vi "Get Timestamp.vi"(8 "error in (no error)":errorcluster, 9 "Data Type (default value)":timestamp, 10 "Offset":i32, 11 "JSON":string) -> (0 "error out":errorcluster, 1 "Timestamp":timestamp, 2 "Offset past match":i32)   [LabVIEW 2017, in "JSONtext.lvlib"]
uses:
  JSONtext.lvlib
  Parsing/Advance past String.vi
  String Subset.vi
  Strip Quotes and Unescape.vi
  Get Number Text.vi
  Parsing/NaN or null to Integer ERROR.vi
  Parsing/Advance past Number.vi
  <vilib>/Utility/error.llb/Error Cluster From Error Code.vi
  Parsing/Parsing Error.vi
  Unescape JSON string.vi
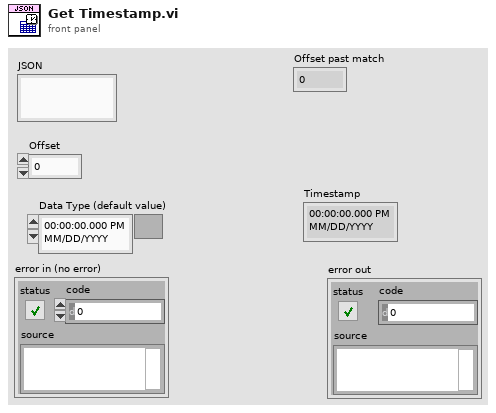
[diagram p1: front panel]
types:
  T1 = typedef "JSONtext.lvlib/Parsing State.ctl" = enum16{"Parser Error", "Object", "Array", "String", "Number/Other", "Leading Whitespace", "Object end", "Array end", "Value end"}
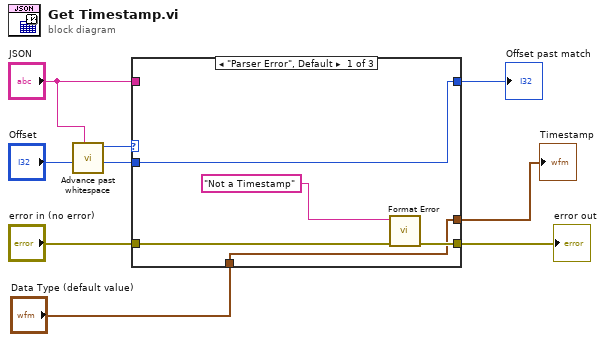
[diagram p0: block diagram]
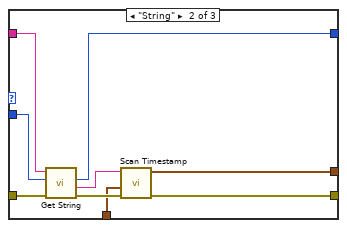
[diagram p2: hidden frame]
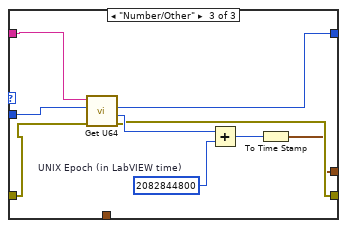
[diagram p3: hidden frame]
diagram:
  n1 = call "Advance past whitespace.vi"("JSON"="JSON", "Offset"="Offset") -> ("Offset of first non-whitespace"=w3:i32, "Parser State"=w2:T1)  [unwired: 8 in]
  n2 = case shown="\"Parser Error\", Default" w2 {
    tunnel: "error in (no error)" -> [w13 w23 w27]
    tunnel: [w11 w20 w25] -> w8
    tunnel: [w14 w19 w26] -> w7
    tunnel: [w12 w18 w24] -> w6
    tunnel: "JSON" -> [_ w17 w32]
    tunnel: w3 -> [w12 w16 w31]
    tunnel: "Data Type (default value)" -> [w11 w15 _]
    frame "Parser Error", Default {
      n3 = call "Format Error.vi"("error in (no error)"=w13, "error message"="Not a Timestamp" ("format string")) -> ("error out"=w14:errorcluster)  [unwired: 9 in]
    }
    frame "String" {
      n4 = call "Get String.vi"("error in (no error)"=w23, "Offset"=w16, "JSON"=w17) -> ("error out"=w22:errorcluster, "String"=w21:string, "Offset past match"=w18:i32)  [unwired: 6 in]
      n5 = call "Scan Timestamp.vi"("error in (no error)"=w22, "default value"=w15, "String"=w21) -> ("error out"=w19:errorcluster, "Timestamp"=w20:timestamp)  [unwired: 7 in]
    }
    frame "Number/Other" {
      w30 = i64 2082844800  # UNIX Epoch (in LabVIEW time)
      n6 = call "Get U64.vi"("error in (no error)"=w27, "Offset"=w31, "JSON"=w32) -> ("error out"=w26:errorcluster, "Number"=w28:u64, "Offset past match"=w24:i32)  [unwired: 6 in]
      n7 = Add(x=w28, y=w30) -> (x+y=w29:u64)
      n8 = To Time Stamp(1:w29) -> (0:w25:timestamp)
    }
  }
  "error out" <- w7
  "Offset past match" <- w6
  "Timestamp" <- w8
